vi "ErrorMessage_IAT.vi"(8 "error in (no error)":errorcluster, 11 "Message":string) -> (0 "error out":errorcluster)   [LabVIEW 2018]
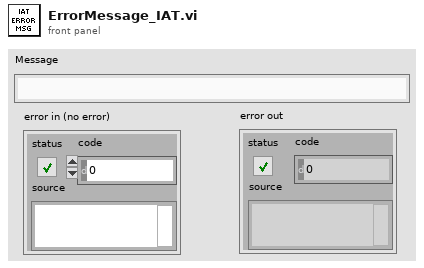
[diagram p1: front panel]
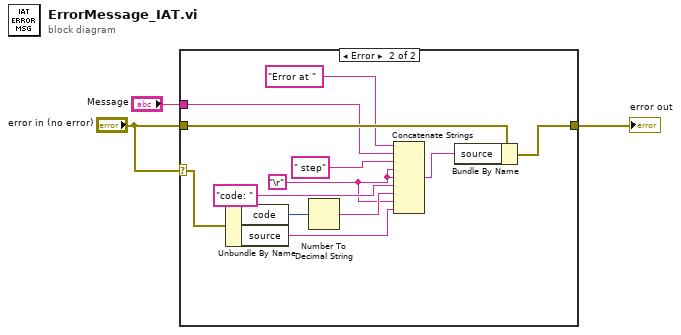
[diagram p0: block diagram]
diagram:
  n1 = case shown="Error" "error in (no error)" {
    selector: "error in (no error)" -> [_ w10]
    tunnel: [w4 w15] -> w1
    tunnel: "error in (no error)" -> [w4 w16]
    tunnel: "Message" -> [_ w12]
    frame No Error {
    }
    frame Error {
      w6 = "\r"
      n2 = Unbundle By Name(w10) -> ("code"=w8:i32, "source"=w5:string)
      n3 = Number To Decimal String(number=w8) -> (decimal integer string=w7:string)  [unwired: 1 in]
      n4 = Concatenate Strings("Error at " ("string"), w12, " step", w6, w6, "code: ", w7, w6, w5) -> (w14:string)
      n5 = Bundle By Name(cluster=w16, "source"=w14) -> (w15:errorcluster)
    }
  }
  "error out" <- w1
